vi "Tree_GetIndexFromTag.vi"(8 "Error In":errorcluster, 10 "Tag IN":string, 11 "Tree Refnum IN":refnum<vi>) -> (0 "Error Out":errorcluster, 2 "Index OUT":i32, 3 "Tree Refnum OUT":refnum<vi>)   [LabVIEW 2012]
doc: "SciScan 1.2 160622"
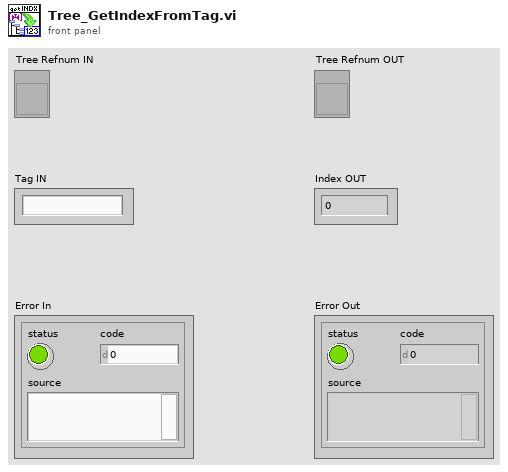
[diagram p1: front panel]
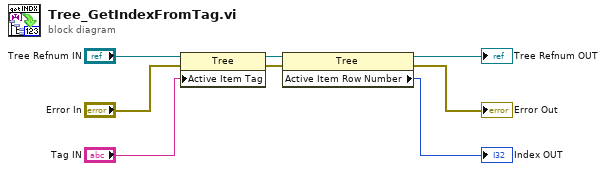
[diagram p0: block diagram]
diagram:
  n1 = property class="Tree"(reference="Tree Refnum IN", error in="Error In", "Active Item Tag"="Tag IN") -> (reference out=w5:refnum<vi>, error out=w4:errorcluster)
  n2 = property class="Tree"(reference=w5, error in=w4) -> (reference out=→"Tree Refnum OUT":refnum<vi>, error out=→"Error Out":errorcluster, "Active Item Row Number"=→"Index OUT":i32)
